vi "transition.vi"(8 "error in (no error)":errorcluster, 10 "Context In":refnum<class "Context.lvclass">, 11 "State in":refnum<class "State.lvclass">) -> (0 "error out":errorcluster, 2 "Context Out":refnum<class "Context.lvclass">, 3 "State out":refnum<class "State.lvclass">)   [LabVIEW 2018, in "State.lvclass"]
uses:
  State.lvclass
  Context/Context.lvclass
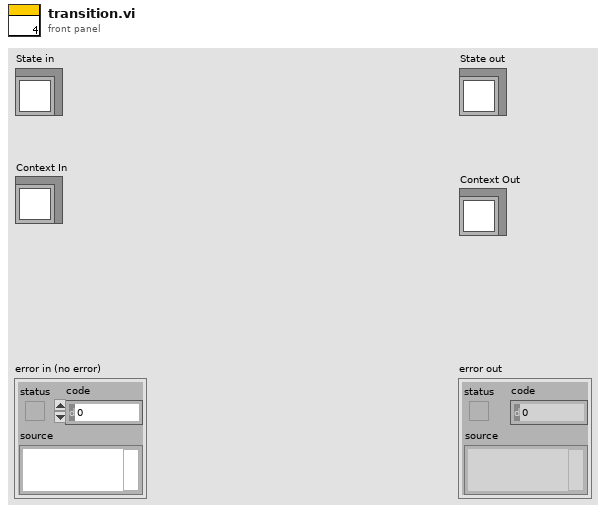
[diagram p1: front panel]
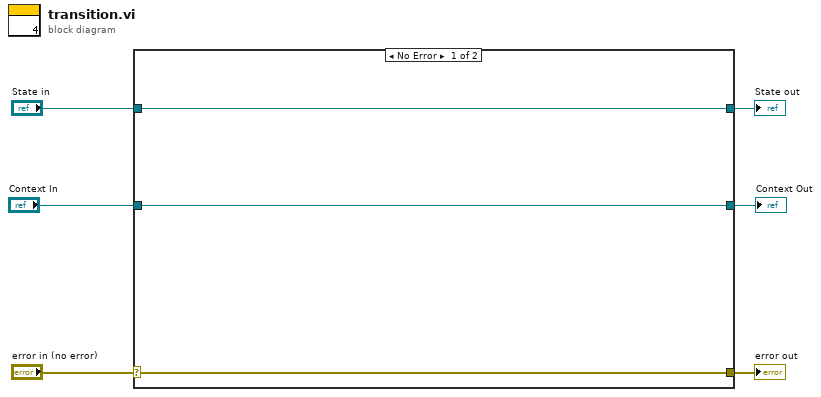
[diagram p0: block diagram]
diagram:
  n1 = case shown="No Error" "error in (no error)" {
    selector: "error in (no error)" -> [w9 w11]
    tunnel: [w9 w11] -> w5
    tunnel: [w7 w12] -> w3
    tunnel: "State in" -> [w7 w12]
    tunnel: [w8 w10] -> w2
    tunnel: "Context In" -> [w8 w10]
    frame No Error {
    }
    frame Error {
      # "Wire the error cluster across even in the \"No Error\"\ncase so that warnings get propagated."
    }
  }
  "error out" <- w5
  "State out" <- w3
  "Context Out" <- w2
